vi "To Proper Case__ogtk.vi"   [LabVIEW 2020]
doc: "Converts alphabetic characters in string to proper case (i.e., first alphabetic character to uppercase, all others to lowercase)."
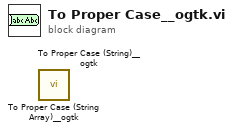
[diagram p0: block diagram]
diagram:
  n1 = call <userlib>:"To Proper Case (String Array)__ogtk.vi"() -> ()  [unwired: 5 in, 1 out]
  n2 = call <userlib>:"To Proper Case (String)__ogtk.vi"() -> ()  [unwired: 5 in, 1 out]
